vi "Add Items by Text Array and SubItems to ListView.vi"(8 "error in (no error)":errorcluster caption="错误输入（无错误）", 9 "SubItems":string[][](array[string]), 10 "Text":string[](array[string]), 11 "ListViewClass 输入":refnum<class "ListViewClass.lvclass"> caption="DNL_LabVIEW Object in") -> (0 "error out":errorcluster caption="错误输出", 3 "ListViewClass 输出":refnum<class "ListViewClass.lvclass"> caption="DNL_LabVIEW Object out")   [LabVIEW 2012, in "ListViewClass.lvclass"]
uses:
  ListViewClass.lvclass
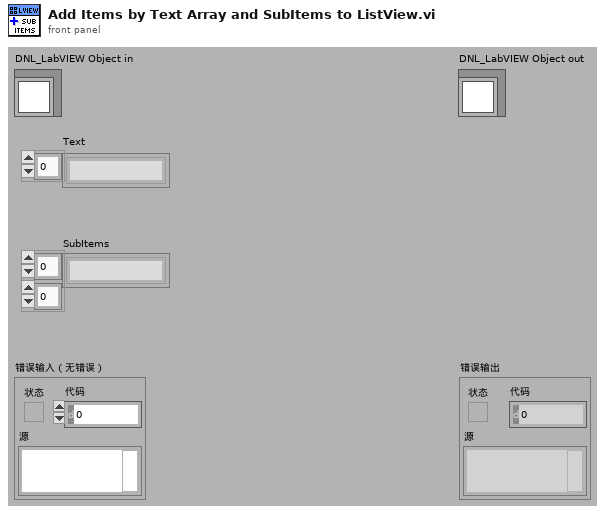
[diagram p1: front panel]
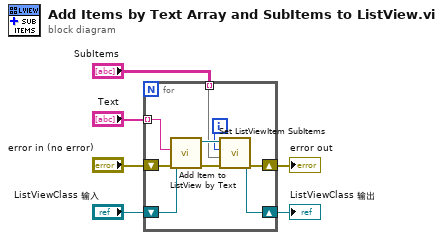
[diagram p0: block diagram]
diagram:
  n1 = for {
    shift-right: [w15] -> w2
    shift-left: "ListViewClass 输入" -> [w12]
    shift-right: [w14] -> w1
    shift-left: "error in (no error)" -> [w10]
    tunnel: "Text" -> [w11] mode=indexing
    tunnel: "SubItems" -> [w7] mode=indexing
    i -> [w8]
    n2 = call "Add Item to ListView by Text.vi"("error in (no error)"=w10, "Text"=w11, "ListViewClass 输入"=w12) -> ("error out"=w9:errorcluster, "ListViewClass 输出"=w13:refnum<class "ListViewClass.lvclass">)  [unwired: 7 in]
    n3 = call "Set ListViewItem SubItems.vi"("error in (no error)"=w9, "SubItems"=w7, "index"=w8, "ListViewClass 输入"=w13) -> ("error out"=w14:errorcluster, "ListViewClass 输出"=w15:refnum<class "ListViewClass.lvclass">)  [unwired: 6 in]
  }
  "error out" <- w1
  "ListViewClass 输出" <- w2
